vi "Thermometer Readout.vi"() -> ()   [LabVIEW 2023]
uses:
  Global Variables/MQM Data Transfer All.vi
  Global Variables/Thermometers.vi
panel:
  out "Global Stop":bool
  out "R_C2 Log Domain":dbl[](array[numeric])
  out "R_C1 Log Domain":dbl[](array[numeric])
  out "R_H Log Domain":dbl[](array[numeric])
  out "R_C2 coeffs":dbl[](array[numeric])
  out "R_C1 coeffs":dbl[](array[numeric])
  out "R_H coeffs":dbl[](array[numeric])
  in  "T_C2 Lockin":enum16{"LI1", "LI2", "LI3"}(ring)=enum."LI3"
  out "I_therm":dbl
  in  "T_C1 Lockin":enum16{"LI1", "LI2", "LI3"}(ring)=enum."LI2"
  in  "T_H Lockin":enum16{"LI1", "LI2", "LI3"}(ring)
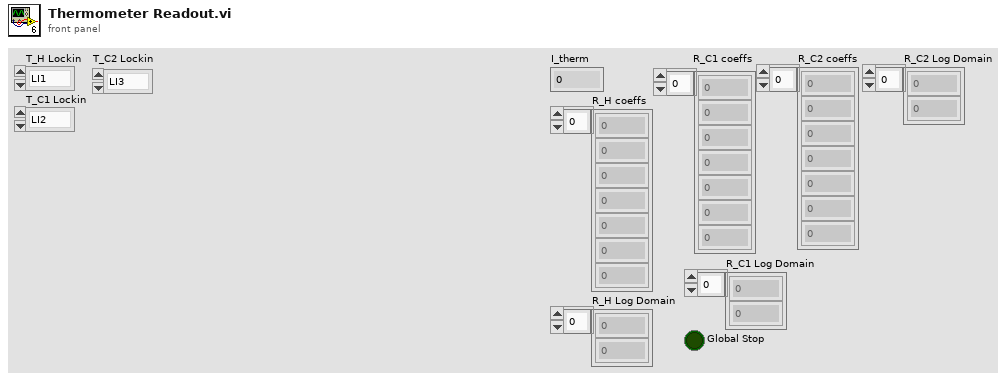
[diagram p1: front panel]
types:
  T1 = typedef "ZI_Frontpanel_All.ctl" = cluster{"Lockin 1 Demod 0":cluster{"R(V)":dbl, "Theta (deg)":dbl, "Timestamp (ms)":u32, "X(V)":dbl, "Y(V)":dbl, "frequency (Hz)":dbl, "output voltage (V)":dbl}, "Lockin 2 Demod 0":cluster{"R(V)":dbl, "Theta (deg)":dbl, "Timestamp (ms)":u32, "X(V)":dbl, "Y(V)":dbl, "frequency (Hz)":dbl, "output voltage (V)":dbl}, "Lockin 3 Demod 0":cluster{"R(V)":dbl, "Theta (deg)":dbl, "Timestamp (ms)":u32, "X(V)":dbl, "Y(V)":dbl, "frequency (Hz)":dbl, "output voltage (V)":dbl}, "Lockin 4 Demod 0":cluster{"R(V)":dbl, "Theta (deg)":dbl, "Timestamp (ms)":u32, "X(V)":dbl, "Y(V)":dbl, "frequency (Hz)":dbl, "output voltage (V)":dbl}, "LI1 active":bool, "LI2 active":bool, "LI3 active":bool, "LI4 active":bool}
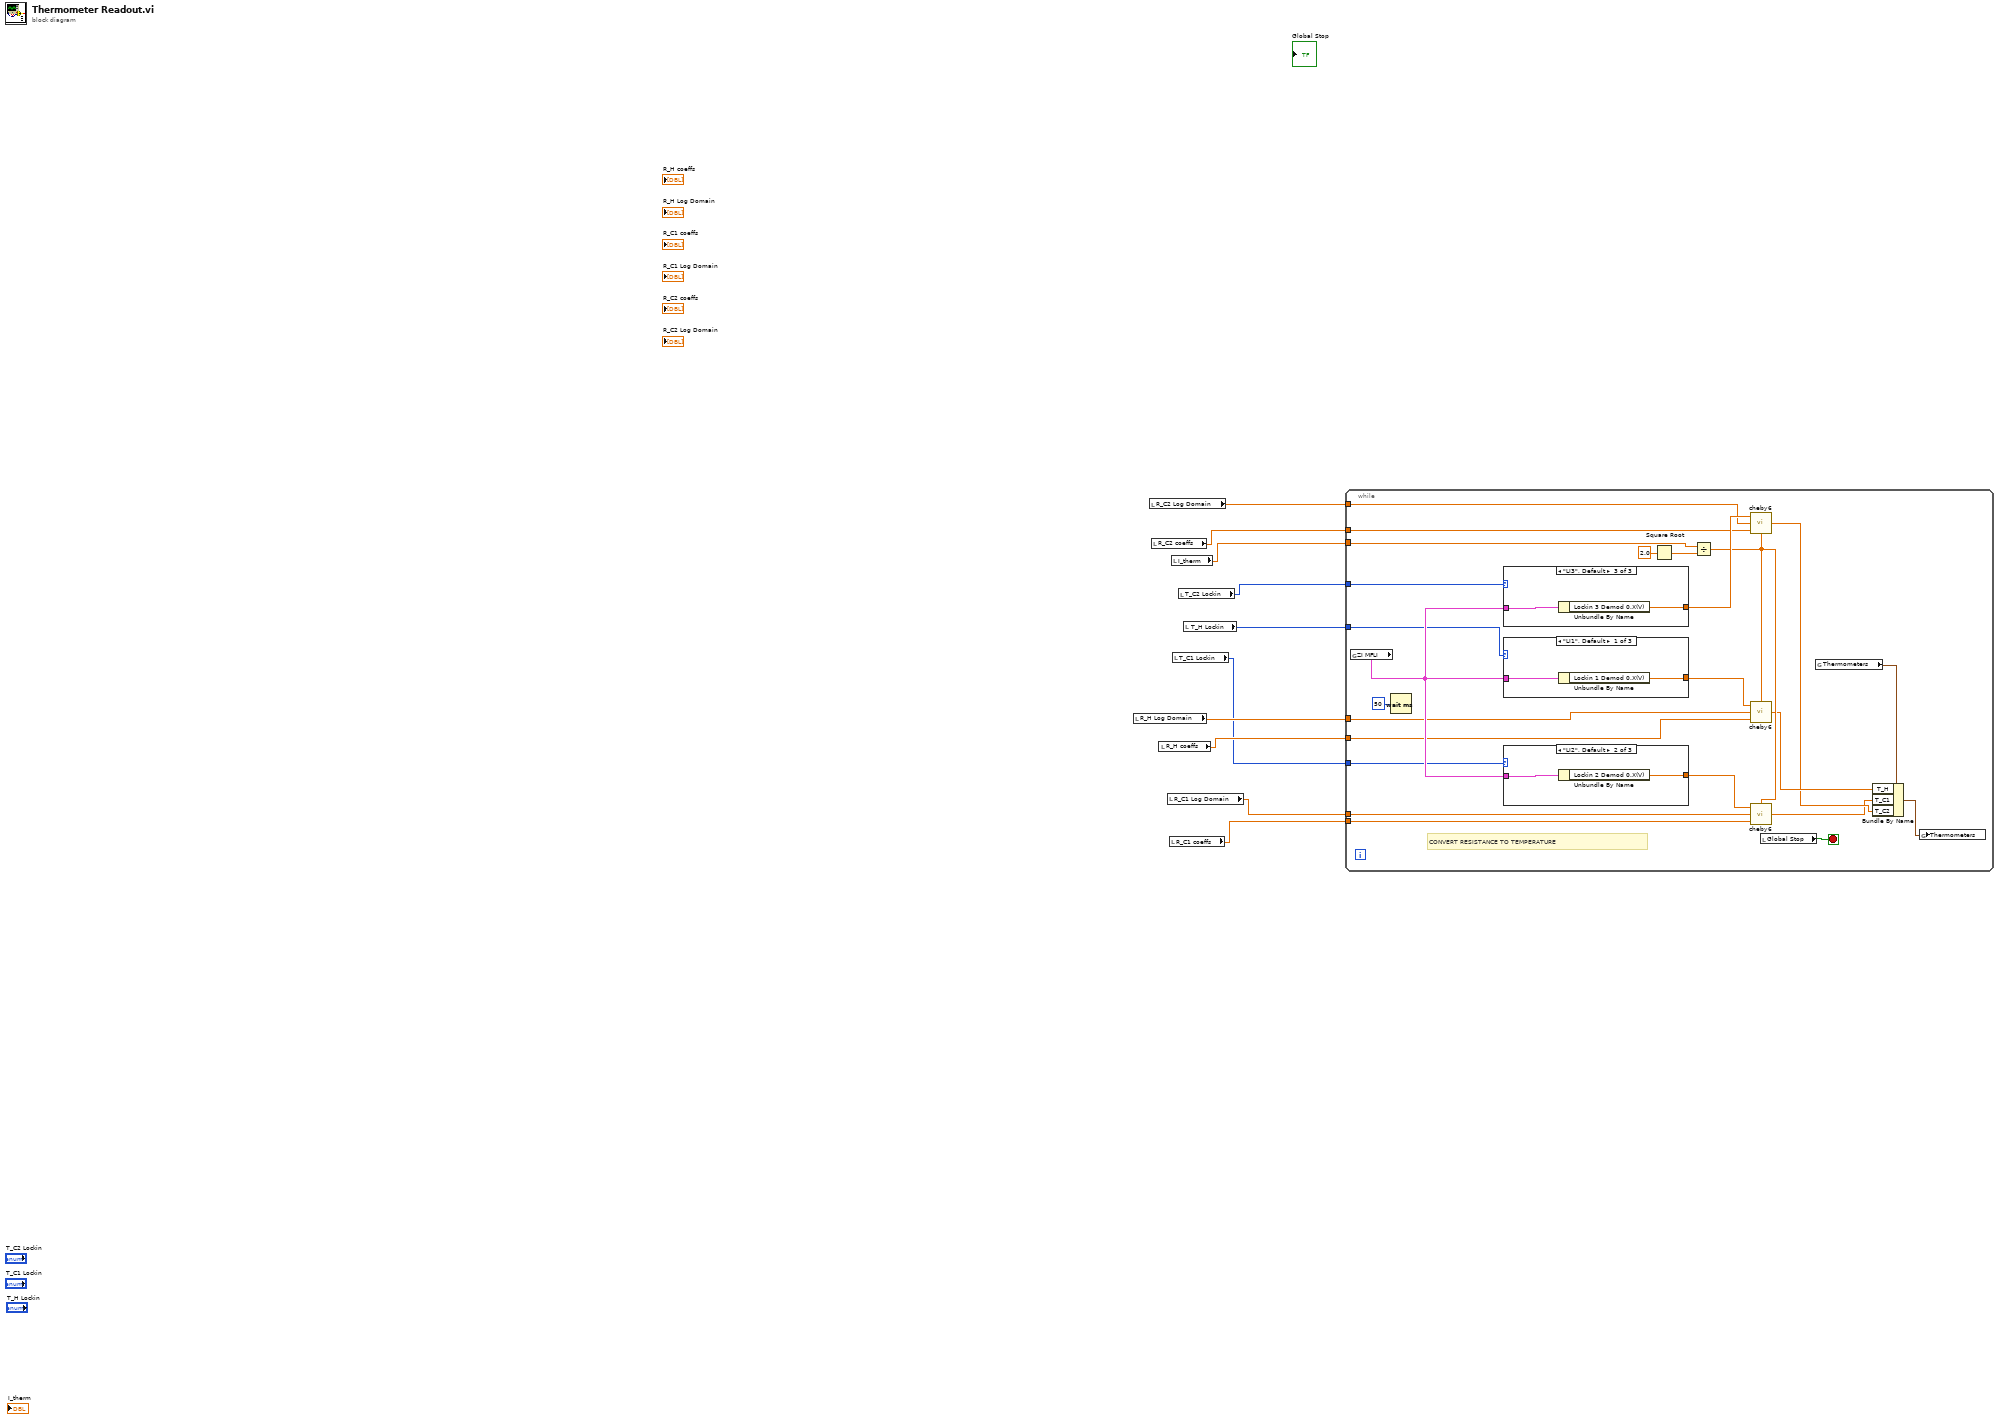
[diagram p0: block diagram]
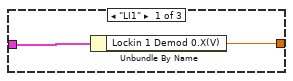
[diagram p2: hidden frame]
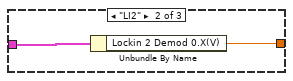
[diagram p3: hidden frame]
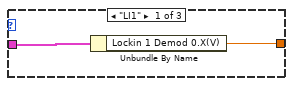
[diagram p4: hidden frame]
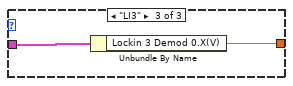
[diagram p5: hidden frame]
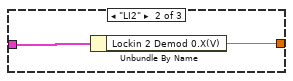
[diagram p6: hidden frame]
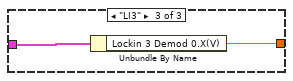
[diagram p7: hidden frame]
diagram:
  n1 = local read "R_H Log Domain"() -> (w8:dbl[])
  n2 = local read "R_C2 Log Domain"() -> (w5:dbl[])
  n3 = local read "R_C2 coeffs"() -> (w6:dbl[])
  n4 = local read "R_H coeffs"() -> (w7:dbl[])
  n5 = local read "R_C1 Log Domain"() -> (w10:dbl[])
  n6 = local read "R_C1 coeffs"() -> (w9:dbl[])
  n7 = local read "I_therm"() -> (w1:dbl)
  n8 = local read "T_C1 Lockin"() -> (w2:enum16{"LI1", "LI2", "LI3"})
  n9 = local read "T_C2 Lockin"() -> (w4:enum16{"LI1", "LI2", "LI3"})
  n10 = local read "T_H Lockin"() -> (w3:enum16{"LI1", "LI2", "LI3"})
  n11 = while {
    tunnel: w10 -> [w26]
    tunnel: w9 -> [w25]
    tunnel: w8 -> [w24]
    tunnel: w7 -> [w23]
    tunnel: w6 -> [w22]
    tunnel: w5 -> [w21]
    tunnel: w4 -> [w20]
    tunnel: w3 -> [w19]
    tunnel: w2 -> [w18]
    tunnel: w1 -> [w17]
    stop <- w28 stop-if-true
    # "CONVERT RESISTANCE TO TEMPERATURE"
    n12 = global read "MQM Data Transfer All.vi" "ZI MFLI"() -> (w27:T1)
    n13 = Wait (ms)(milliseconds to wait=u32 50) -> ()  [unwired: 1 out]
    n14 = case shown="\"LI3\", Default" w20 {
      tunnel: w27 -> [w36 w37 w40]
      tunnel: [w35 w38 w39] -> w30
      frame "LI1" {
        n15 = Unbundle By Name(w36) -> ("Lockin 1 Demod 0.X(V)"=w35:dbl)
      }
      frame "LI2" {
        n16 = Unbundle By Name(w37) -> ("Lockin 2 Demod 0.X(V)"=w38:dbl)
      }
      frame "LI3", Default {
        n17 = Unbundle By Name(w40) -> ("Lockin 3 Demod 0.X(V)"=w39:dbl)
      }
    }
    n18 = case shown="\"LI1\", Default" w19 {
      tunnel: w27 -> [w48 w49 w52]
      tunnel: [w47 w50 w51] -> w32
      frame "LI1", Default {
        n19 = Unbundle By Name(w48) -> ("Lockin 1 Demod 0.X(V)"=w47:dbl)
      }
      frame "LI2" {
        n20 = Unbundle By Name(w49) -> ("Lockin 2 Demod 0.X(V)"=w50:dbl)
      }
      frame "LI3" {
        n21 = Unbundle By Name(w52) -> ("Lockin 3 Demod 0.X(V)"=w51:dbl)
      }
    }
    n22 = case shown="\"LI2\", Default" w18 {
      tunnel: w27 -> [w42 w44 w46]
      tunnel: [w41 w43 w45] -> w31
      frame "LI1" {
        n23 = Unbundle By Name(w42) -> ("Lockin 1 Demod 0.X(V)"=w41:dbl)
      }
      frame "LI2", Default {
        n24 = Unbundle By Name(w44) -> ("Lockin 2 Demod 0.X(V)"=w43:dbl)
      }
      frame "LI3" {
        n25 = Unbundle By Name(w46) -> ("Lockin 3 Demod 0.X(V)"=w45:dbl)
      }
    }
    n26 = Square Root(x=2.0) -> (sqrt(x)=w34:dbl)
    n27 = Divide(x=w17, y=w34) -> (x/y=w29:dbl)
    n28 = call "cheby6.vi"("I"=w29, "Coefs"=w22, "RU/L"=w21, "LIX"=w30) -> ("T"=w14:dbl)
    n29 = call "cheby6.vi"("I"=w29, "Coefs"=w23, "RU/L"=w24, "LIX"=w32) -> ("T"=w15:dbl)
    n30 = call "cheby6.vi"("I"=w29, "Coefs"=w25, "RU/L"=w26, "LIX"=w31) -> ("T"=w13:dbl)
    n31 = local read "Global Stop"() -> (w28:bool)
    n32 = global read "Thermometers.vi" "Thermometers"() -> (w16:cluster{"T_H":dbl, "T_C1":dbl, "T_C2":dbl})
    n33 = Bundle By Name(cluster=w16, "T_H"=w15, "T_C1"=w13, "T_C2"=w14) -> (w12:cluster{"T_H":dbl, "T_C1":dbl, "T_C2":dbl})
    n34 = global write "Thermometers.vi" "Thermometers"(w12) -> ()
  }
